vi "Set Class Wire Pens.vi"() -> ()   [LabVIEW 2013]
panel:
  in  "Hue":u32(colorbox)
  in  "Color":enum16{"Wire Pens", "Icon Header", "Hue"}(ring)
  in  "Color Picker Array":u32[][](array[colorbox])=[[16777215, 0, 15658209, 2050429, 5210557, 12603469, 10206041, 8414370, 4959430, 16225862], [15921906, 8355711, 14539203, 13031920, 14411249, 15916251, 15462877, 15065324, 14413555, 16640730], [14211288, 5855577, 12893591, 9286626, 12111076, 15055287, 14148540, 13418969, 12049896, 16504245], [12566463, 4144959, 9668947, 5541332, 9810903, 14259860, 12834459, 11707079, 9620956, 16433295], [10855845, 2500134, 4801577, 1521245, 3563666, 9778996, 7770684, 6244730, 3245467, 14904329], [8355711, 789516, 1907472, 992318, 2375777, 6497315, 5202216, 4141393, 2119783, 9914374], [12582912, 16711680, 16760832, 16776960, 9621584, 45136, 45296, 28864, 8288, 7352480]]
  in  "Picture":picture
  in  "Wire Pens":T1(array[cluster])=[{"Foreground Color"=2375777, "Background Color"=9810903, "Fill Pattern"={"Row 0"=0, "Row 1"=0, "Row 2"=0, "Row 3"=0, "Row 4"=0, "Row 5"=0, "Row 6"=0, "Row 7"=0}, "Width"=3, "Mode"=enum."Copy", "Style"=enum."Solid", "Fill Rule"=enum."Even Odd", "End Caps"=enum."Default"}, {"Foreground Color"=2375777, "Background Color"=14411249, "Fill Pattern"={"Row 0"=0, "Row 1"=0, "Row 2"=0, "Row 3"=0, "Row 4"=0, "Row 5"=0, "Row 6"=0, "Row 7"=0}, "Width"=5, "Mode"=enum."Copy", "Style"=enum."Solid", "Fill Rule"=enum."Even Odd", "End Caps"=enum."Default"}] {"Fill Pattern"."Row 0" format="%08b"; "Fill Pattern"."Row 1" format="%08b"; "Fill Pattern"."Row 2" format="%08b"; "Fill Pattern"."Row 3" format="%08b"; "Fill Pattern"."Row 4" format="%08b"; "Fill Pattern"."Row 5" format="%08b"; "Fill Pattern"."Row 6" format="%08b"; "Fill Pattern"."Row 7" format="%08b"}
  in  "Type":T2(ring)
  in  "Path":path
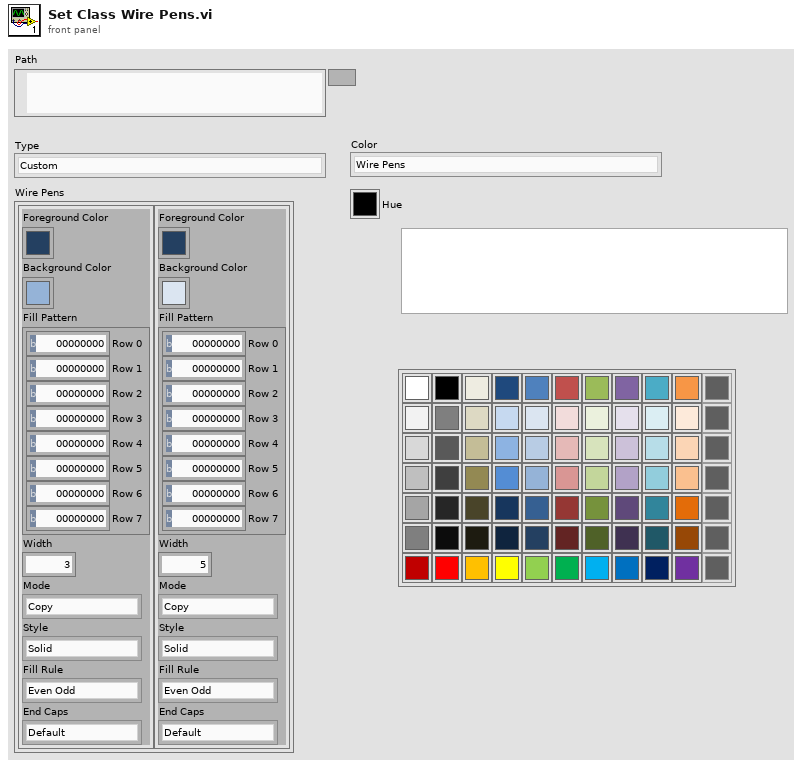
[diagram p1: front panel]
types:
  T1 = cluster{"Foreground Color":u32, "Background Color":u32, "Fill Pattern":cluster{"Row 0":u8, "Row 1":u8, "Row 2":u8, "Row 3":u8, "Row 4":u8, "Row 5":u8, "Row 6":u8, "Row 7":u8}, "Width":i16, "Mode":enum16{"Copy", "Or", "Exclusive Or", "Bit Clear", "Not Copy", "Not Or", "Nor Exclusive Or", "Not Bit Clear"}, "Style":enum32{"Solid", "Dash", "Dot", "Dash Dot", "Dash Dot Dot"}, "Fill Rule":enum32{"Even Odd", "Winding"}, "End Caps":enum32{"Default", "Flat"}}[]
  T2 = enum16{"Custom", "FTW Rope", "FTW Chain", "Chevron", "Test"}
  T3 = cluster{"Foreground Color":u32, "Background Color":u32, "Fill Pattern":cluster{"Row 0":u8, "Row 1":u8, "Row 2":u8, "Row 3":u8, "Row 4":u8, "Row 5":u8, "Row 6":u8, "Row 7":u8}, "Width":i16, "Mode":enum16{"Copy", "Or", "Exclusive Or", "Bit Clear", "Not Copy", "Not Or", "Nor Exclusive Or", "Not Bit Clear"}, "Style":enum32{"Solid", "Dash", "Dot", "Dash Dot", "Dash Dot Dot"}, "Fill Rule":enum32{"Even Odd", "Winding"}, "End Caps":enum32{"Default", "Flat"}}
  T4 = enum32{"invalid VI type", "Standard VI", "Control VI", "Global VI", "Polymorphic VI", "Configuration VI", "SubSystem", "Facade VI", "Method VI", "Statechart Diagram VI"}
  T5 = typedef "imagedata.ctl" = cluster{"image type":i32, "image depth":i32, "image":u8[], "mask":u8[], "colors":u32[], "Rectangle":cluster{"left":i16, "top":i16, "right":i16, "bottom":i16}}
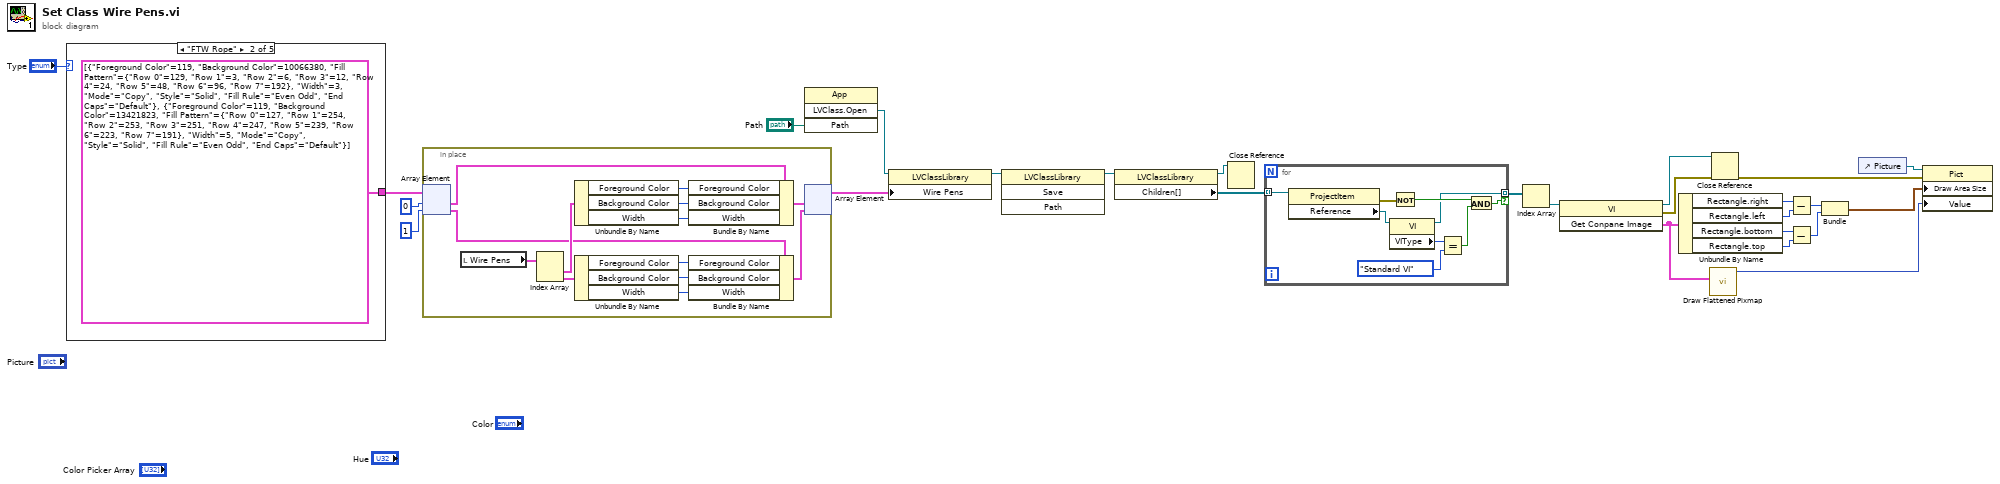
[diagram p0: block diagram]
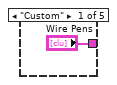
[diagram p2: hidden frame]
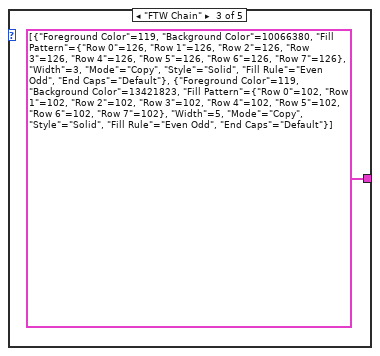
[diagram p3: hidden frame]
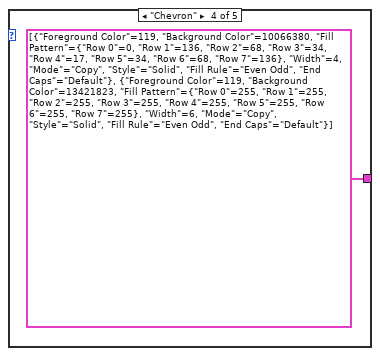
[diagram p4: hidden frame]
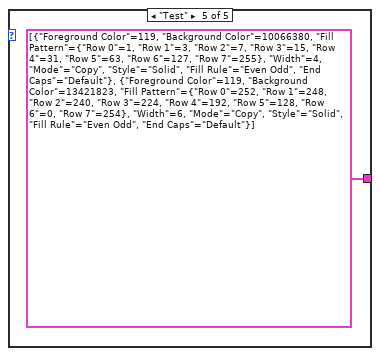
[diagram p5: hidden frame]
diagram:
  n1 = case shown="\"FTW Rope\"" "Type" {
    tunnel: ["Wire Pens" T1 [{"Foreground Color"=119, "Background Color"=10066380, "Fill Pattern"={"Row 0"=129, "Row 1"=3, "Row 2"=6, "Row 3"=12, "Row 4"=24, "Row 5"=48, "Row 6"=96, "Row 7"=192}, "Width"=3, "Mode"=enum."Copy", "Style"=enum."Solid", "Fill Rule"=enum."Even Odd", "End Caps"=enum."Default"}, {"Foreground Color"=119, "Background Color"=13421823, "Fill Pattern"={"Row 0"=127, "Row 1"=254, "Row 2"=253, "Row 3"=251, "Row 4"=247, "Row 5"=239, "Row 6"=223, "Row 7"=191}, "Width"=5, "Mode"=enum."Copy", "Style"=enum."Solid", "Fill Rule"=enum."Even Odd", "End Caps"=enum."Default"}] ("Array") T1 [{"Foreground Color"=119, "Background Color"=10066380, "Fill Pattern"={"Row 0"=126, "Row 1"=126, "Row 2"=126, "Row 3"=126, "Row 4"=126, "Row 5"=126, "Row 6"=126, "Row 7"=126}, "Width"=3, "Mode"=enum."Copy", "Style"=enum."Solid", "Fill Rule"=enum."Even Odd", "End Caps"=enum."Default"}, {"Foreground Color"=119, "Background Color"=13421823, "Fill Pattern"={"Row 0"=102, "Row 1"=102, "Row 2"=102, "Row 3"=102, "Row 4"=102, "Row 5"=102, "Row 6"=102, "Row 7"=102}, "Width"=5, "Mode"=enum."Copy", "Style"=enum."Solid", "Fill Rule"=enum."Even Odd", "End Caps"=enum."Default"}] ("Array") T1 [{"Foreground Color"=119, "Background Color"=10066380, "Fill Pattern"={"Row 0"=0, "Row 1"=136, "Row 2"=68, "Row 3"=34, "Row 4"=17, "Row 5"=34, "Row 6"=68, "Row 7"=136}, "Width"=4, "Mode"=enum."Copy", "Style"=enum."Solid", "Fill Rule"=enum."Even Odd", "End Caps"=enum."Default"}, {"Foreground Color"=119, "Background Color"=13421823, "Fill Pattern"={"Row 0"=255, "Row 1"=255, "Row 2"=255, "Row 3"=255, "Row 4"=255, "Row 5"=255, "Row 6"=255, "Row 7"=255}, "Width"=6, "Mode"=enum."Copy", "Style"=enum."Solid", "Fill Rule"=enum."Even Odd", "End Caps"=enum."Default"}] ("Array") T1 [{"Foreground Color"=119, "Background Color"=10066380, "Fill Pattern"={"Row 0"=1, "Row 1"=3, "Row 2"=7, "Row 3"=15, "Row 4"=31, "Row 5"=63, "Row 6"=127, "Row 7"=255}, "Width"=4, "Mode"=enum."Copy", "Style"=enum."Solid", "Fill Rule"=enum."Even Odd", "End Caps"=enum."Default"}, {"Foreground Color"=119, "Background Color"=13421823, "Fill Pattern"={"Row 0"=252, "Row 1"=248, "Row 2"=240, "Row 3"=224, "Row 4"=192, "Row 5"=128, "Row 6"=0, "Row 7"=254}, "Width"=6, "Mode"=enum."Copy", "Style"=enum."Solid", "Fill Rule"=enum."Even Odd", "End Caps"=enum."Default"}] ("Array")] -> w22
    frame "Custom" {
    }
    frame "FTW Rope" {
    }
    frame "FTW Chain" {
    }
    frame "Chevron" {
    }
    frame "Test" {
    }
  }
  n2 = in-place {
    n3 = in-place-array #1(w22, 0, 1) -> (w44:T3, w36:T3)
    n4 = local read "Wire Pens"() -> (w43:T1)
    n5 = Index Array(array=w43) -> (element #1=w42:T3, element #2=w38:T3)  [unwired: 2 in]
    n6 = Unbundle By Name(w42) -> ("Foreground Color"=w41:u32, "Background Color"=w35:u32, "Width"=w33:i16)
    n7 = Unbundle By Name(w38) -> ("Foreground Color"=w39:u32, "Background Color"=w34:u32, "Width"=w32:i16)
    n8 = Bundle By Name(cluster=w44, "Foreground Color"=w41, "Background Color"=w35, "Width"=w33) -> (w40:T3)
    n9 = Bundle By Name(cluster=w36, "Foreground Color"=w39, "Background Color"=w34, "Width"=w32) -> (w37:T3)
    n10 = in-place-array #1(w40, w37) -> (w21:T1)  [unwired: 2 out]
  }
  n11 = invoke class="App" method="LVClass.Open"("Path"="Path") -> ("LVClass.Open"=w24:refnum<vi>)  [unwired: 3 in, 3 out]
  n12 = property class="LVClassLibrary"(reference=w24, "Wire Pens"=w21) -> (reference out=w23:refnum<vi>)  [unwired: 1 in, 1 out]
  n13 = invoke class="LVClassLibrary" method="Save"(reference=w23) -> (reference out=w3:refnum<vi>)  [unwired: 3 in, 3 out]
  n14 = property class="LVClassLibrary"(reference=w3) -> (reference out=w1:refnum<vi>, "Children[]"=w2:refnum<vi>[])  [unwired: 1 in, 1 out]
  n15 = Close Reference(reference=w1) -> ()  [unwired: 1 in, 1 out]
  n16 = for {
    tunnel: w2 -> [w53] mode=indexing
    tunnel: [w49] -> w5 mode=indexing if=w46
    n17 = property class="ProjectItem"(reference=w53) -> (error out=w51:errorcluster, "Reference"=w52:refnum<vi>)  [unwired: 1 in, 1 out]
    n18 = property class="VI"(reference=w52) -> (reference out=w49:refnum<vi>, "VIType"=w48:T4)  [unwired: 1 in, 1 out]
    n19 = Not(x=w51) -> (.not. x?=w50:bool)
    n20 = Equal?(x=w48, y=T4."Standard VI") -> (x = y?=w45:bool)
    n21 = And(x=w50, y=w45) -> (x .and. y?=w46:bool)
  }
  n22 = Index Array(array=w5) -> (element=w4:refnum<vi>)  [unwired: 1 in]
  n23 = invoke class="VI" method="Get Conpane Image"(reference=w4) -> (reference out=w17:refnum<vi>, error out=w18:errorcluster, "Get Conpane Image"=w7:T5)  [unwired: 2 in]
  n24 = Unbundle By Name(w7) -> ("Rectangle.right"=w15:i16, "Rectangle.left"=w14:i16, "Rectangle.bottom"=w13:i16, "Rectangle.top"=w12:i16)
  n25 = call <vilib>:"Draw Flattened Pixmap.vi"("image data"=w7) -> ("new picture"=w8:picture)  [unwired: 8 in]
  n26 = Close Reference(reference=w17, error in (no error)=w18) -> (error out=w16:errorcluster)
  n27 = Subtract(x=w15, y=w14) -> (x-y=w11:i16)
  n28 = Subtract(x=w13, y=w12) -> (x-y=w10:i16)
  n29 = Bundle(w11, w10) -> (w6:cluster{i16, i16})  [unwired: 1 in]
  n30 = control-ref of="Picture"() -> (w9:refnum<vi>)
  n31 = property class="Pict"(reference=w9, error in=w16, "Draw Area Size"=w6, "Value"=w8) -> ()  [unwired: 2 out]
